vi "Create File Path Type.vi"(2 "PATH Only?":bool, 3 "File Type":string(combo)=".ini", 4 "Filename-Description":string, 5 "Timestamp?":bool, 6 "Folder Name":string, 7 "Serial #":string) -> (1 "File Path":path)   [LabVIEW 2025]
doc: "Creates folder in default data directory. If the folder already exists, it does nothing."
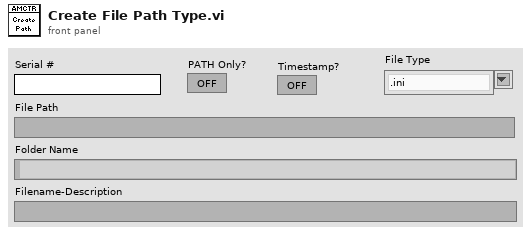
[diagram p1: front panel]
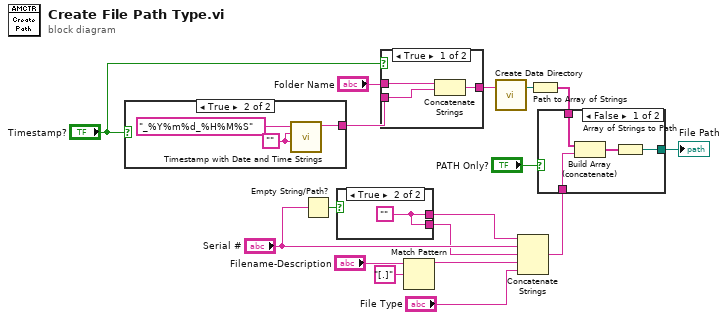
[diagram p0: block diagram]
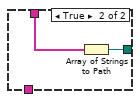
[diagram p2: hidden frame]
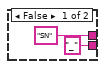
[diagram p4: hidden frame]
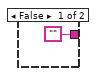
[diagram p5: hidden frame]
diagram:
  n1 = case shown="True" "Timestamp?" {
    tunnel: ["" w19] -> w4
    frame False {
    }
    frame True {
      w21 = ""
      n2 = call "Timestamp with Date and Time Strings.vi"("Delimiter (Time)"=w21, "Delimiter (Date)"=w21, "Timestamp Format String"="_%Y%m%d_%H%M%S" ("time format string (%c)")) -> ("Timestamp String"=w19:string)  [unwired: 6 in, 2 out]
    }
  }
  n3 = Empty String/Path?(string/path="Serial #") -> (empty?=w11:bool)
  n4 = case shown="True" w11 {
    tunnel: ["SN" ("string") w24] -> w17
    tunnel: ["_" w24] -> w7
    frame False {
    }
    frame True {
      w24 = ""
    }
  }
  n5 = case shown="True" "Timestamp?" {
    tunnel: [w26 w28] -> w3
    tunnel: "Folder Name" -> [w27 w28]
    tunnel: w4 -> [w25 _]
    frame True {
      n6 = Concatenate Strings(w27, w25) -> (w26:string)
    }
    frame False {
    }
  }
  n7 = Match Pattern(string="Filename-Description", regular expression="[.]" ("search string")) -> (before substring=w10:string)  [unwired: 1 in, 3 out]
  n8 = call "Create Data Directory.vi"("Folder Name"=w3) -> ("Path"=w5:path)  [unwired: 2 in]
  n9 = Concatenate Strings(w17, "Serial #", w7, w10, "File Type") -> (w8:string)
  n10 = Path to Array of Strings(0:w5) -> (2:w2:string[])  [unwired: 1 out]
  n11 = case shown="False" "PATH Only?" {
    tunnel: [w31 w34] -> w16
    tunnel: w8 -> [w30 _]
    tunnel: w2 -> [w29 w33]
    frame False {
      n12 = Build Array (concatenate)(w29, w30) -> (w32:string[])
      n13 = Array of Strings to Path(0:w32) -> (2:w31:path)  [unwired: 1 in]
    }
    frame True {
      n14 = Array of Strings to Path(0:w33) -> (2:w34:path)  [unwired: 1 in]
    }
  }
  "File Path" <- w16
